vi "ALLPROPS20_Test.vi"(8 "error in (no error)":errorcluster) -> (0 "error out 2":errorcluster caption="error out", 3 "Passed?":bool)   [LabVIEW 2016]
panel:
  out "Inputs":T1={"hOut"="T,P,D,H,E,S", "iUnits"=0, "iMass"=5, "iFlag"=0, "T"=100.0, "D"=0.179, "z"=[1.0]}
  in  "Fluid of interest":string="HELIUM.FLD"
  out "Outputs":T2
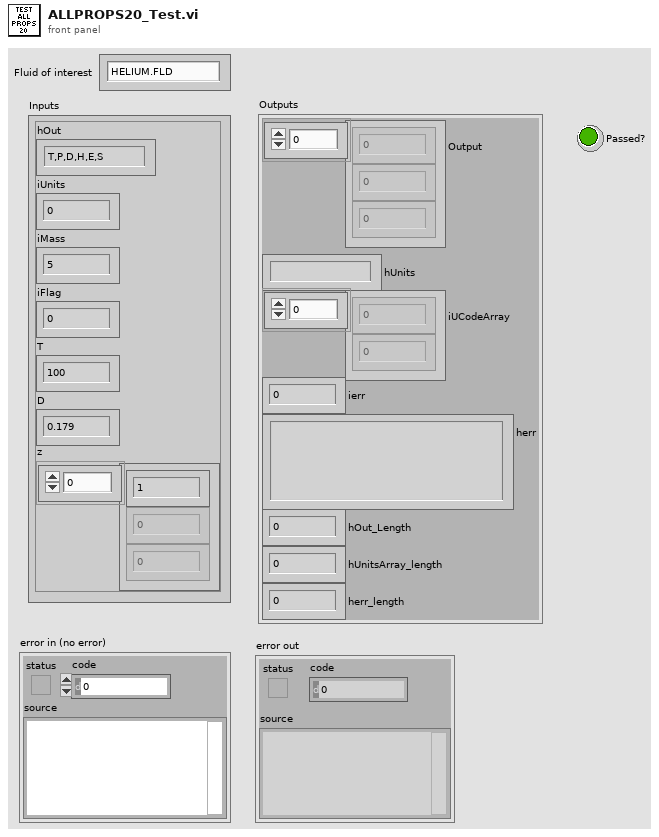
[diagram p1: front panel]
types:
  T1 = cluster{"hOut":string, "iUnits":i32, "iMass":i32, "iFlag":i32, "T":dbl, "D":dbl, "z":dbl[]}
  T2 = cluster{"Output":dbl[], "hUnits":string, "iUCodeArray":i32[], "ierr":i32, "herr":string, "hOut_Length":i32, "hUnitsArray_length":i32, "herr_length":i32}
  T3 = typedef "Mixture Composition cluster_d.ctl" = cluster{"Mixture Name":string, "Molecular weight (g/mol)":dbl, "Critical temperature (K)":dbl, "Critical Pressure (kPa)":dbl, "Critical Density (mol/L)":dbl, "# Components":i32, "Fluid File Paths":path[], "Component molar fractions":dbl[], "Refprop Main Directory":path, "DLL Version Number":dbl}
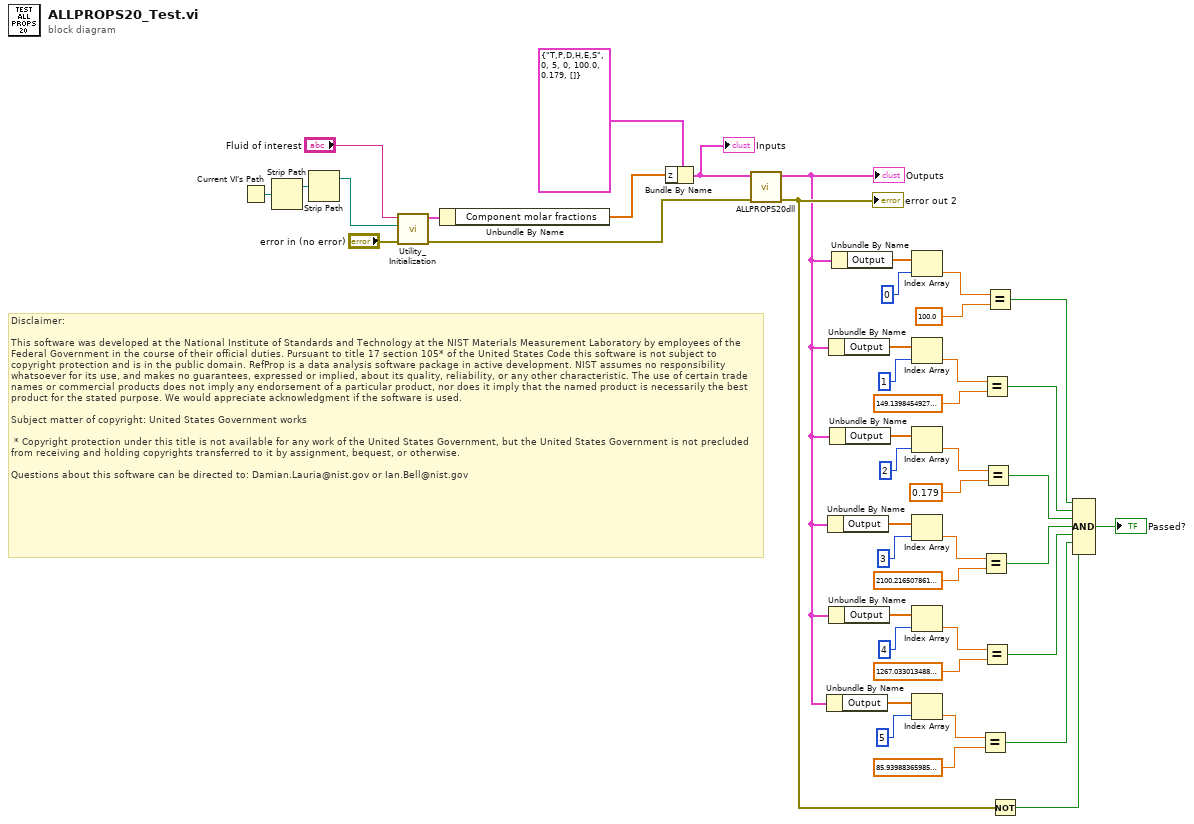
[diagram p0: block diagram]
diagram:
  # "Disclaimer:\n\nThis software was developed at the National Institute of Standards and Technology at the NIST Materials Measurement Laboratory by employees of the Federal Government in the course of their official duties. Pursuant to title 17 section 105* of the United States Code this software is not subject to copyright protection and is in the public domain. RefProp is a data analysis software package in active development. NIST assumes no responsibility whatsoever for its use, and makes no guarantees, expressed or implied, about its quality, reliability, or any other characteristic. The use of certain trade names or commercial products does not imply any endorsement of a particular product, nor does it imply that the named product is necessarily the best product for the stated purpose. We would appreciate acknowledgment if the software is used.\n \nSubject matter of copyright: United States Government works\n  \n * Copyright protection under this title is not available for any work of the United States Government, but the United States Government is not precluded from receiving and holding copyrights transferred to it by assignment, bequest, or otherwise.\n\nQuestions about this software can be directed to: Damian.Lauria@nist.gov or Ian.Bell@nist.gov"
  n1 = Current VI's Path() -> (path=w42:path)
  n2 = Strip Path(path=w42) -> (stripped path=w41:path)  [unwired: 1 out]
  n3 = Strip Path(path=w41) -> (stripped path=w40:path)  [unwired: 1 out]
  n4 = call "Utility_Initialization.vi"("error in (no error)"="error in (no error)", "path"=w40, "Fluidofinterest"="Fluid of interest") -> ("error out"=w32:errorcluster, "Mixure Cluster out"=w39:T3)  [unwired: 6 in, 1 out]
  n5 = Unbundle By Name(w39) -> ("Component molar fractions"=w44:dbl[])
  n6 = Bundle By Name(cluster=T1 {"hOut"="T,P,D,H,E,S", "iUnits"=0, "iMass"=5, "iFlag"=0, "T"=100.0, "D"=0.179, "z"=[]} ("Inputs"), "z"=w44) -> (w31:T1)
  "Inputs" <- w31
  n7 = call "ALLPROPS20dll.vi"("error in (no error)"=w32, "Inputs"=w31) -> ("error out"=w33:errorcluster, "Outputs"=w14:T2)  [unwired: 8 in]
  "Outputs" <- w14
  "error out 2" <- w33
  n8 = Unbundle By Name(w14) -> ("Output"=w16:dbl[])
  n9 = Unbundle By Name(w14) -> ("Output"=w23:dbl[])
  n10 = Unbundle By Name(w14) -> ("Output"=w28:dbl[])
  n11 = Unbundle By Name(w14) -> ("Output"=w19:dbl[])
  n12 = Unbundle By Name(w14) -> ("Output"=w26:dbl[])
  n13 = Unbundle By Name(w14) -> ("Output"=w36:dbl[])
  n14 = Index Array(array=w36, index=0) -> (element=w35:dbl)
  n15 = Index Array(array=w28, index=1) -> (element=w5:dbl)
  n16 = Index Array(array=w26, index=2) -> (element=w25:dbl)
  n17 = Index Array(array=w23, index=3) -> (element=w22:dbl)
  n18 = Index Array(array=w19, index=4) -> (element=w18:dbl)
  n19 = Index Array(array=w16, index=5) -> (element=w15:dbl)
  n20 = Equal?(x=w15, y=85.93988365985514 ("element 5")) -> (x = y?=w8:bool)
  n21 = Equal?(x=w22, y=2100.216507861462 ("element")) -> (x = y?=w10:bool)
  n22 = Equal?(x=w5, y=149.13984549271007 ("element")) -> (x = y?=w12:bool)
  n23 = Equal?(x=w18, y=1267.0330134887802 ("element 4")) -> (x = y?=w9:bool)
  n24 = Equal?(x=w25, y=0.179 ("element 2")) -> (x = y?=w11:bool)
  n25 = Equal?(x=w35, y=100.0 ("element")) -> (x = y?=w13:bool)
  n26 = Not(x=w33) -> (.not. x?=w7:bool)
  n27 = Compound Arithmetic op=AND(w13, w12, w11, w10, w9, w8, w7) -> (→"Passed?":bool)
